vi "Read Msg Pattern.vi"(8 "error in (no error)":errorcluster, 11 "Generic Logger in":refnum<class "Generic Logger.lvclass">) -> (0 "error out":errorcluster, 2 "Msg Pattern":string, 3 "Generic Logger out":refnum<class "Generic Logger.lvclass">)   [LabVIEW 2020, in "Logging.lvlib" / "Generic Logger.lvclass"]
uses:
  Generic Logger.lvclass
  Generic Logger.lvclass/Generic Logger.ctl
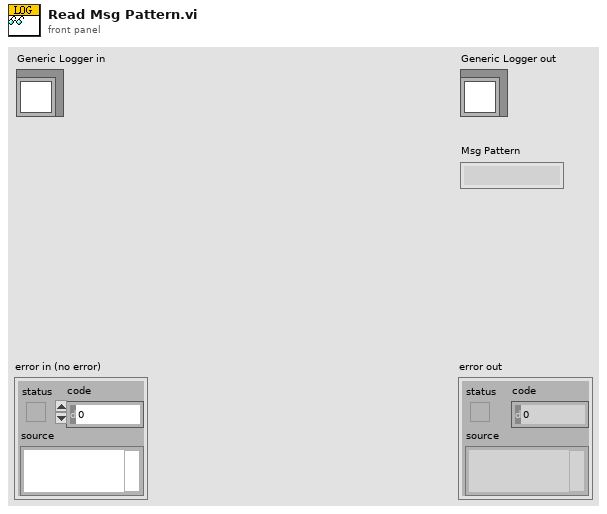
[diagram p1: front panel]
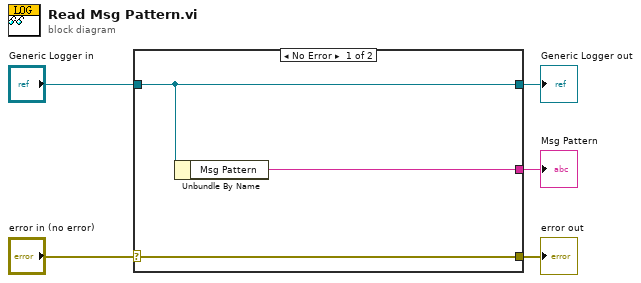
[diagram p0: block diagram]
diagram:
  n1 = case shown="No Error" "error in (no error)" {
    selector: "error in (no error)" -> [w8 w9]
    tunnel: [w8 w9] -> w4
    tunnel: [w7 w10] -> w2
    tunnel: "Generic Logger in" -> [w7 w10]
    tunnel: [w6 _] -> w1
    frame No Error {
      n2 = Unbundle By Name(w7) -> ("Msg Pattern"=w6:string)
    }
    frame Error {
    }
  }
  "error out" <- w4
  "Generic Logger out" <- w2
  "Msg Pattern" <- w1
